vi "Read SDI Value.vi"(8 "error in":errorcluster, 11 "32-bit word in":refnum<class "32-bit Word.lvclass">) -> (0 "error out":errorcluster, 2 "SDI value":u8=2 format="%02b", 3 "32-bit word out":refnum<class "32-bit Word.lvclass">)   [LabVIEW 2020, in "32-bit Word.lvclass"]
uses:
  32-bit Word.lvclass
  32-bit Word.lvclass/32-bit Word.ctl
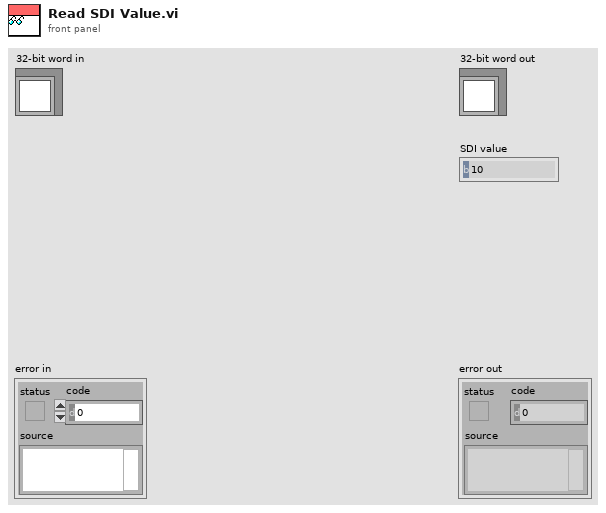
[diagram p1: front panel]
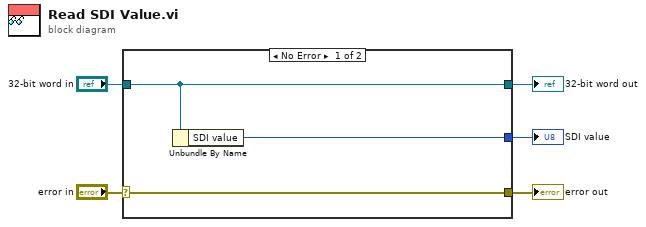
[diagram p0: block diagram]
diagram:
  n1 = case shown="No Error" "error in" {
    selector: "error in" -> [w8 w9]
    tunnel: [w8 w9] -> w4
    tunnel: [w7 w10] -> w2
    tunnel: "32-bit word in" -> [w7 w10]
    tunnel: [w6 _] -> w1
    frame No Error {
      n2 = Unbundle By Name(w7) -> ("SDI value"=w6:u8)
    }
    frame Error {
    }
  }
  "error out" <- w4
  "32-bit word out" <- w2
  "SDI value" <- w1
